vi "NI VeriStand - Get Custom Device Driver.vi"(8 "error in (no error)":errorcluster, 11 "Device Ref in":T4 format="%.0x") -> (0 "error out":errorcluster, 1 "Driver VI Path (Host)":T1, 2 "Driver VI Path (RT)":path, 3 "Device Ref out":T4 format="%.0x", 5 "Execution mode":T3)   [LabVIEW 2020, in "Custom Device API.lvlib"]
doc: "Returns information about the execution mode and driver VI paths for a custom device."
uses:
  <vilib>/NI VeriStand/Custom Device API/Custom Device API.lvlib
  <vilib>/NI VeriStand/Custom Device API/Custom Device Item Ref.ctl
  <vilib>/NI VeriStand/Custom Device API/Custom Device Execution Mode.ctl
  <vilib>/NI VeriStand/Custom Device API/Path Specification.ctl
  <vilib>/NI VeriStand/Custom Device API/Path Type.ctl
  2555c4fe-586f-4302-8689-911da6d0a91f.vi
  <vilib>/NI VeriStand/Custom Device API/Custom Device Offline Path.vi
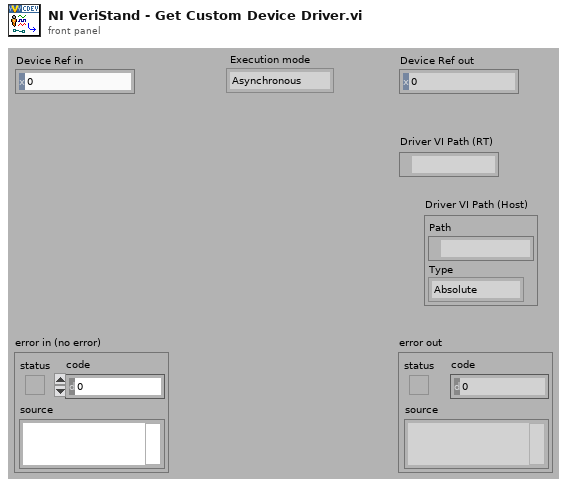
[diagram p1: front panel]
types:
  T1 = typedef "Custom Device API.lvlib/Path Specification.ctl" = cluster{"Path":path, "Type":T2}
  T2 = typedef "Custom Device API.lvlib/Path Type.ctl" = enum16{"Absolute", "To Base", "To Common Data Dir", "To Application Data Dir"}
  T3 = typedef "Custom Device API.lvlib/Custom Device Execution Mode.ctl" = enum16{"Asynchronous", "Inline HW Interface", "Inline Model Interface", "Inline Timing and Sync", "Asynchronous Timing and Sync"}
  T4 = typedef "Custom Device API.lvlib/Custom Device Item Ref.ctl" = u64
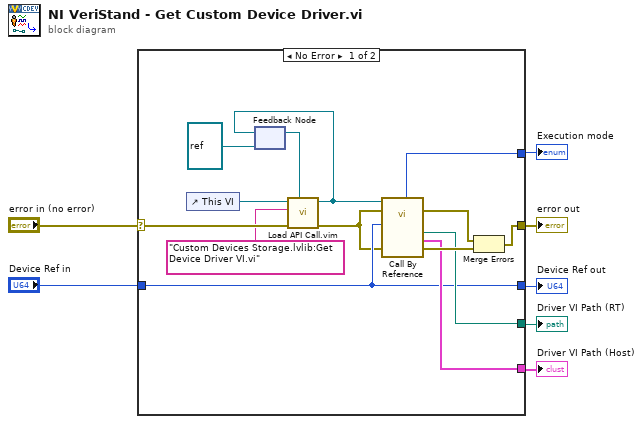
[diagram p0: block diagram]
diagram:
  n1 = case shown="No Error" "error in (no error)" {
    selector: "error in (no error)" -> [w13 w23]
    tunnel: [w20 w23] -> w7
    tunnel: "Device Ref in" -> [w16 w22]
    tunnel: [w16 w22] -> w5
    tunnel: [w19 _] -> w4
    tunnel: [w18 _] -> w3
    tunnel: [w17 _] -> w2
    frame No Error {
      n2 = control-ref of="This VI"() -> (w14:refnum<vi>)
      n3 = feedback #1(refnum<vi> refnum ("type specifier VI Refnum (for type only)")) -> (w15:refnum<vi>)
      n4 = call "Load API Call.vim"("VI reference in"=w15, "error in (no error)"=w13, "VI qualified name"="Custom Devices Storage.lvlib:Get Device Driver VI.vi", "Caller VI ref"=w14) -> ("error out"=w11:errorcluster, "VI reference"=w12:refnum<vi>)  [unwired: 6 in]
      n5 = feedback-in #1(w12) -> ()
      n6 = call-by-ref "?"(reference=w12, error in=w11, 8:"error in (no error)"=w11, "Device Ref in"=w16) -> (error out=w8:errorcluster, 0:"error out"=w21:errorcluster, "Driver VI Path (Host)"=w17:T1, "Driver VI Path (RT)"=w18:path, "Executon mode"=w19:T3)  [unwired: 5 in, 2 out]
      n7 = Merge Errors(w8, w21) -> (w20:errorcluster)
    }
    frame Error {
    }
  }
  "Device Ref out" <- w5
  "error out" <- w7
  "Driver VI Path (RT)" <- w3
  "Execution mode" <- w4
  "Driver VI Path (Host)" <- w2
